vi "Updater Mass Split PI TDMS Files.vi"(8 "error in (no error)":errorcluster, 11 "Spartan TDM Path":path) -> (0 "error out":errorcluster)   [LabVIEW 2011]
uses:
  Summitek EXT/OpenG EXT/file/file.llb/Strip Path Extension - Path__ogtk.vi
panel:
  out "file names":string[](array[string])
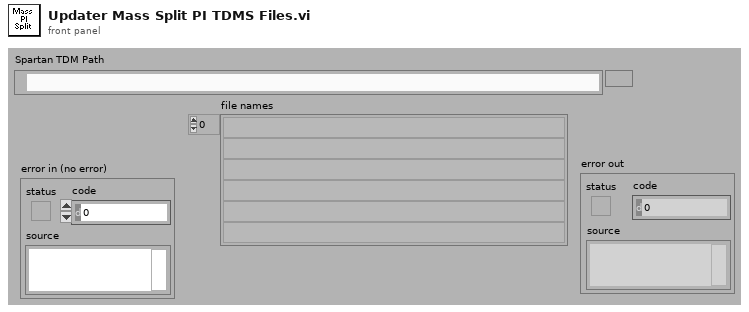
[diagram p1: front panel]
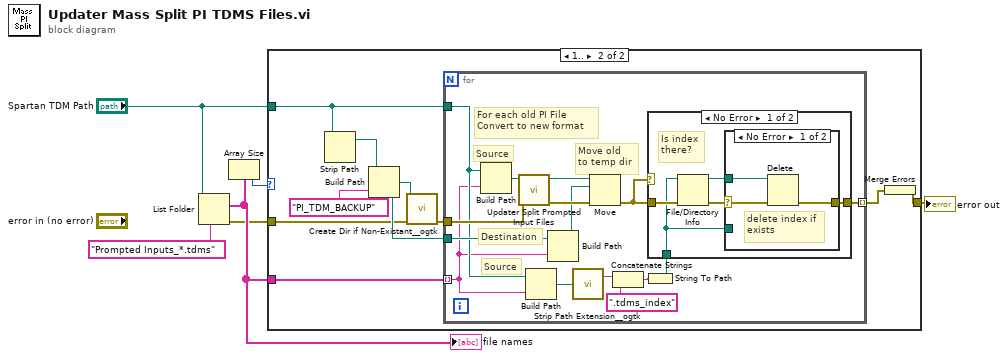
[diagram p0: block diagram]
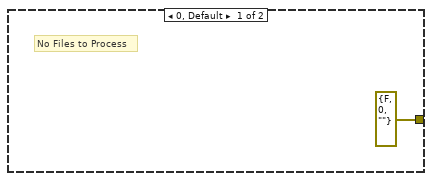
[diagram p2: hidden frame]
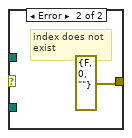
[diagram p3: hidden frame]
diagram:
  n1 = List Folder(path="Spartan TDM Path", pattern="Prompted Inputs_*.tdms") -> (filenames=w3:string[], error out=w1:errorcluster)  [unwired: 1 in, 3 out]
  "file names" <- w3
  n2 = Array Size(array=w3) -> (size(s)=w2:i32)
  n3 = case shown="1.." w2 {
    tunnel: w3 -> [_ w16]
    tunnel: "Spartan TDM Path" -> [_ w13]
    tunnel: [errorcluster {"status"=FALSE, "code"=0, "source"=""} ("error out") w10] -> w4
    tunnel: w1 -> [_ w8]
    frame 0, Default {
      # "No Files to Process"
    }
    frame 1.. {
      n4 = Strip Path(path=w13) -> (stripped path=w12:path)  [unwired: 1 out]
      n5 = Build Path(base path=w12, name or relative path="PI_TDM_BACKUP" ("pattern")) -> (appended path=w14:path)
      n6 = call "Create Dir if Non-Existant__ogtk.vi"("error in (no error)"=w8, "Directory Path"=w14) -> ("error out"=w9:errorcluster)  [unwired: 1 in, 8 out]
      n7 = for {
        tunnel: w13 -> [w20]
        tunnel: w16 -> [w19] mode=indexing
        tunnel: w14 -> [w21]
        tunnel: w9 -> [w28]
        tunnel: [w26] -> w11 mode=indexing
        # "Move old\nto temp dir"
        # "For each old PI File\nConvert to new format"
        # "Destination"
        # "Source"
        # "Source"
        n8 = Build Path(base path=w20, name or relative path=w19) -> (appended path=w31:path)
        n9 = call "Updater Split Prompted Input Files.vi"("error in (no error)"=w28, "source file path (*.tdms)"=w31) -> ("error out"=w29:errorcluster, "source file path (*.tdms) out"=w30:path)  [unwired: 8 out]
        n10 = Build Path(base path=w20, name or relative path=w19) -> (appended path=w18:path)
        n11 = Build Path(base path=w21, name or relative path=w19) -> (appended path=w27:path)
        n12 = call-poly "Strip Path Extension__ogtk.vi"("path"=w18) -> ("root"=w25:string)  [unwired: 1 out]
        n13 = Move(source path=w30, error in=w29, 10:w27) -> (error out=w17:errorcluster)  [unwired: 4 out]
        n14 = Concatenate Strings(w25, ".tdms_index" ("pattern")) -> (w23:string)
        n15 = String To Path(string=w23) -> (path=w22:path)
        n16 = case shown="No Error" w17 {
          tunnel: [w36 w41] -> w26
          tunnel: w17 -> [w35 w41]
          tunnel: w22 -> [w34 _]
          frame No Error {
            # "Is index \nthere?"
            n17 = File/Directory Info(path=w34, error in=w35) -> (path out=w32:path, error out=w33:errorcluster)  [unwired: 5 out]
            n18 = case shown="No Error" w33 {
              selector: w33 -> [w39 _]
              tunnel: [w37 errorcluster {"status"=FALSE, "code"=0, "source"=""} ("error out")] -> w36
              tunnel: w34 -> [_ _]
              tunnel: w32 -> [w38 _]
              frame No Error {
                # "delete index if \nexists"
                n19 = Delete(path (use dialog)=w38, error in=w39) -> (error out=w37:errorcluster)  [unwired: 5 out]
              }
              frame Error {
                # "index does not\nexist"
              }
            }
          }
          frame Error {
            # "Pass through errors\nwith processing"
          }
        }
      }
      n20 = Merge Errors(w11) -> (w10:errorcluster)
    }
  }
  "error out" <- w4
